vi "Data Edge Trigger 4 Samples.vi"(9 "Trigger Level":i16, 11 "Data In":u64) -> (3 "Trigger":bool)   [LabVIEW 2015]
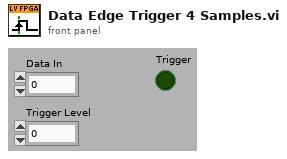
[diagram p1: front panel]
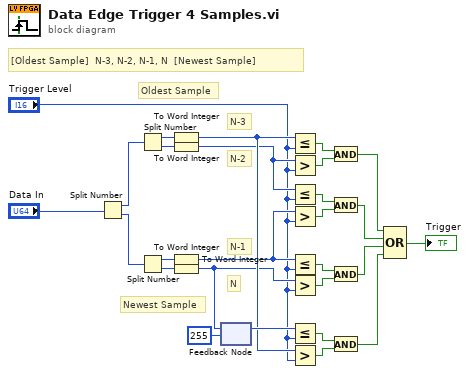
[diagram p0: block diagram]
diagram:
  # "N"
  # "N-1"
  # "N-2"
  # "N-3"
  # "Oldest Sample"
  # "Newest Sample"
  # "[Oldest Sample]  N-3, N-2, N-1, N  [Newest Sample]"
  n1 = Split Number(x="Data In") -> (hi(x)=w27:u32, lo(x)=w26:u32)
  n2 = Split Number(x=w27) -> (hi(x)=w8:u16, lo(x)=w12:u16)
  n3 = Split Number(x=w26) -> (hi(x)=w11:u16, lo(x)=w10:u16)
  n4 = To Word Integer(number=w8) -> (16bit integer=w7:i16)
  n5 = To Word Integer(number=w12) -> (16bit integer=w6:i16)
  n6 = To Word Integer(number=w11) -> (16bit integer=w5:i16)
  n7 = To Word Integer(number=w10) -> (16bit integer=w4:i16)
  n8 = feedback #1(i16 255) -> (w9:i16)
  n9 = feedback-in #1(w4) -> ()
  n10 = Less Or Equal?(x=w7, y="Trigger Level") -> (x <= y?=w24:bool)
  n11 = Greater?(x=w6, y="Trigger Level") -> (0:w25:bool)
  n12 = Less Or Equal?(x=w6, y="Trigger Level") -> (x <= y?=w23:bool)
  n13 = Greater?(x=w5, y="Trigger Level") -> (0:w22:bool)
  n14 = Less Or Equal?(x=w5, y="Trigger Level") -> (x <= y?=w19:bool)
  n15 = Greater?(x=w4, y="Trigger Level") -> (0:w18:bool)
  n16 = Less Or Equal?(x=w9, y="Trigger Level") -> (x <= y?=w20:bool)
  n17 = Greater?(x=w7, y="Trigger Level") -> (0:w21:bool)
  n18 = And(x=w24, y=w25) -> (x .and. y?=w17:bool)
  n19 = And(x=w23, y=w22) -> (x .and. y?=w16:bool)
  n20 = And(x=w19, y=w18) -> (x .and. y?=w15:bool)
  n21 = And(x=w20, y=w21) -> (x .and. y?=w14:bool)
  n22 = Compound Arithmetic op=OR(w17, w16, w15, w14) -> (→"Trigger":bool)
